vi "DP-Init Level.vi"(0 "Multipliers (2D)":dbl[](array[numeric]), 1 "StimGen Out":T3, 2 "DP Freqs":T1, 3 "DataAcq in":T2, 5 "Gains (2D)":dbl[](array[numeric]), 7 "AO Channels":i32[](array[numeric]), 11 "error in (no error)":errorcluster) -> (15 "error out":errorcluster)   [LabVIEW 2020]
uses:
  Typedefs/DP-StimGen.ctl
  Typedefs/DP-DataAcq.ctl
  Typedefs/DP-Freqs.ctl
  PXI DAQ VIs/TDT VIs/TDT-Signal Bank Action.ctl
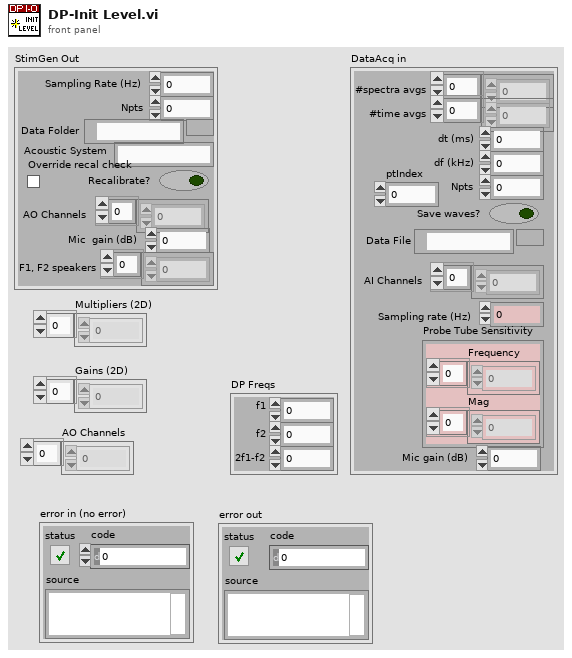
[diagram p1: front panel]
types:
  T1 = typedef "DP-Freqs.ctl" = cluster{"f1":dbl, "f2":dbl, "2f1-f2":dbl}
  T2 = typedef "DP-DataAcq.ctl" = cluster{"#spectra avgs":i32[], "#time avgs":i32[], "dt (ms)":dbl, "df (kHz)":dbl, "Npts":i32, "Save waves?":bool, "Data File":path, "AI Channels":u16[], "Sampling rate (Hz)":dbl, "Probe Tube Sensitivity":cluster{"Frequency":dbl[], "Mag":dbl[]}, "Mic gain (dB)":dbl, "ptIndex":i32}
  T3 = typedef "DP-StimGen.ctl" = cluster{"Sampling Rate (Hz)":dbl, "Npts":i32, "Data Folder":path, "Acoustic System":string, "Recalibrate?":bool, "AO Channels":i32[], "Mic  gain (dB)":dbl, "F1, F2 speakers":i32[], "Override recal check":bool}
  T4 = typedef "TDT-Signal Bank Action.ctl" = enum16{"Init", "Write", "Read", "Rewrite", "Reset", "Recycle", "Ramp up", "Ramp down", "Zero"}
  T5 = typedef "TDT-Device Config.ctl" = cluster{"Output":T6, "Input":T8}
  T6 = typedef "TDT-Output source.ctl" = cluster{"Device":T7, "Num":i32}
  T7 = typedef "TDT-Device ID.ctl" = enum16{"None", "PA5", "RP2", "RL2", "RA16", "RV8", "RX5", "RX6", "RX7", "RX8", "RZ2", "RZ5", "RZ6"}
  T8 = typedef "TDT-Input source.ctl" = enum16{"Front Panel", "RA4LI", "RA16LI"}
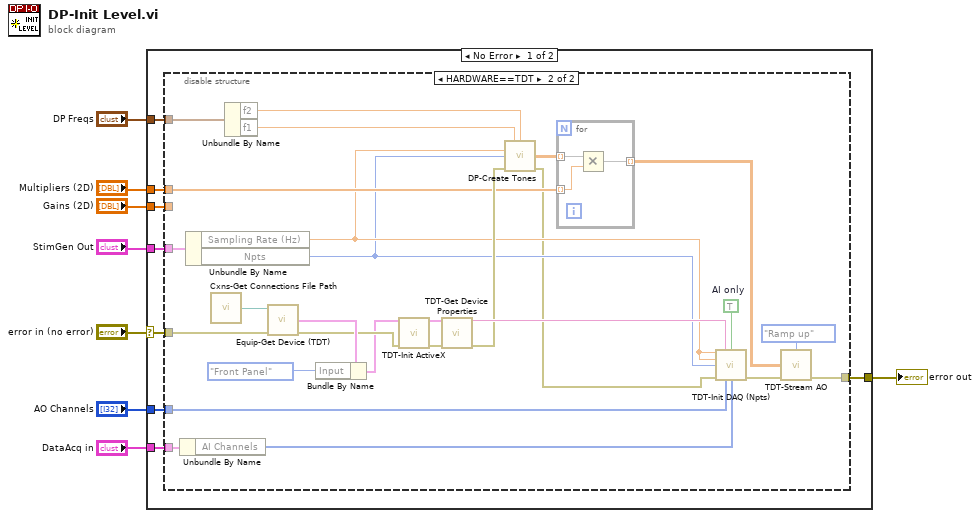
[diagram p0: block diagram]
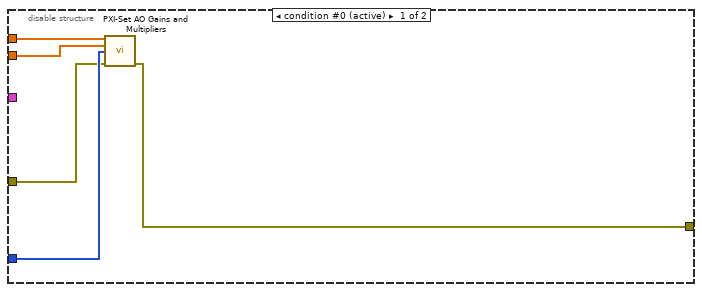
[diagram p2: hidden frame]
diagram:
  n1 = case shown="No Error" "error in (no error)" {
    selector: "error in (no error)" -> [w12 w52]
    tunnel: "AO Channels" -> [w16 _]
    tunnel: [w15 w52] -> w7
    tunnel: "Gains (2D)" -> [w14 _]
    tunnel: "Multipliers (2D)" -> [w13 _]
    tunnel: "DP Freqs" -> [w11 _]
    tunnel: "StimGen Out" -> [w10 _]
    tunnel: "DataAcq in" -> [w9 _]
    frame No Error {
      n2 = disable-structure shown="HARDWARE==TDT" {
        disable-tunnel: w16 -> [w21 w30]
        disable-tunnel: [w20 w26] -> w15
        disable-tunnel: w14 -> [w19 _]
        disable-tunnel: w13 -> [w18 w35]
        disable-tunnel: w12 -> [w17 w34]
        disable-tunnel: w11 -> [_ w41]
        disable-tunnel: w10 -> [_ w38]
        disable-tunnel: w9 -> [_ w29]
        frame condition #0 (active) {
          n3 = call "PXI-Set AO Gains and Multipliers.vi"("Multipliers"=w18, "Gains"=w19, "AO Channels"=w21, "error in (no error)"=w17) -> ("error out"=w20:errorcluster)  [unwired: 11 in]
        }
        frame condition #1 {
          w47 = TRUE  # AI only
          n4 = Unbundle By Name(w29) -> ("AI Channels"=w28:u16[])
          n5 = Unbundle By Name(w38) -> ("Sampling Rate (Hz)"=w33:dbl, "Npts"=w32:i32)
          n6 = call "Cxns-Get Connections File Path.vi"() -> ("Path Out"=w43:path)  [unwired: 1 in]
          n7 = Unbundle By Name(w41) -> ("f2"=w40:dbl, "f1"=w39:dbl)
          n8 = call "Equip-Get Device (TDT).vi"("Path In"=w43, "error in (no error)"=w34) -> ("TDT-Device Config"=w44:T5, "error out"=w23:errorcluster)  [unwired: 11 in, 1 out]
          n9 = Bundle By Name(cluster=w44, "Input"=enum16{"Front Panel", "RA4LI", "RA16LI"}."Front Panel") -> (w22:T5)
          n10 = call "TDT-Init ActiveX.vi"("TDT-Device Config"=w22, "error in (no error)"=w23) -> ("TDT-Device Config out"=w25:T5, "error out"=w24:errorcluster)  [unwired: 10 in, 2 out]
          n11 = call "TDT-Get Device Properties.vi"("TDT-Device Config"=w25, "error in (no error)"=w24) -> ("Circuit File"=w46:string, "error out"=w37:errorcluster)  [unwired: 8 in, 4 out]
          n12 = call "DP-Create Tones.vi"("f1"=w39, "f2"=w40, "Sampling rate (Hz)"=w33, "Npts"=w32, "error in (no error)"=w37) -> ("stimuli"=w36:dbl[][], "error out"=w31:errorcluster)  [unwired: 9 in]
          n13 = for {
            tunnel: [w51] -> w27 mode=indexing
            tunnel: w36 -> [w50] mode=indexing
            tunnel: w35 -> [w49] mode=indexing
            n14 = Multiply(x=w50, y=w49) -> (x*y=w51:dbl[])
          }
          n15 = call "TDT-Init DAQ (Npts).vi"("AO Fs (Hz)"=w33, "Circuit"=w46, "AI only"=w47, "AI Fs (Hz)"=w33, "Num AO Pts"=w32, "error in (no error)"=w31, "AO Channels"=w30, "AI Channels"=w28) -> ("error out"=w48:errorcluster)  [unwired: 3 in, 4 out]
          n16 = call "TDT-Stream AO.vi"("Action"=TDT-Signal_Bank_Action."Ramp up", "Output array"=w27, "error in (no error)"=w48) -> ("error out"=w26:errorcluster)  [unwired: 12 in]
        }
      }
    }
    frame Error {
    }
  }
  "error out" <- w7
